vi "Write to Data Source.vi"(8 "error in (no error)":errorcluster, 11 "Projects in":refnum<class "Projects.lvclass">) -> (0 "error out":errorcluster, 3 "Projects out":refnum<class "Projects.lvclass">)   [LabVIEW 2020, in "Projects.lvclass"]
doc: "Write the data currently in the Project class data to the data source.\n\n03/2025 Erich Schlieper"
uses:
  Projects.lvclass
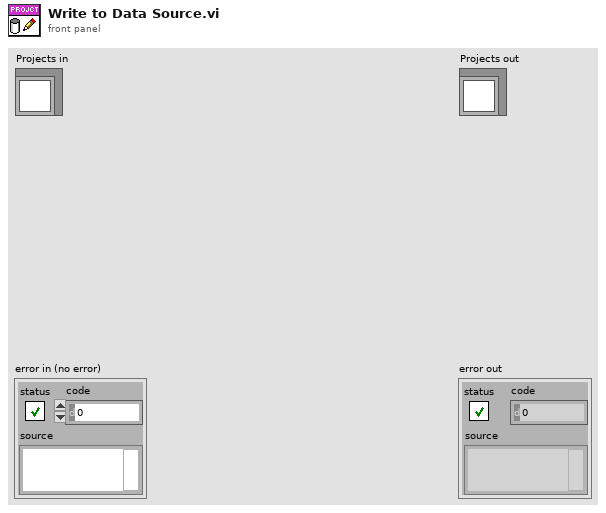
[diagram p1: front panel]
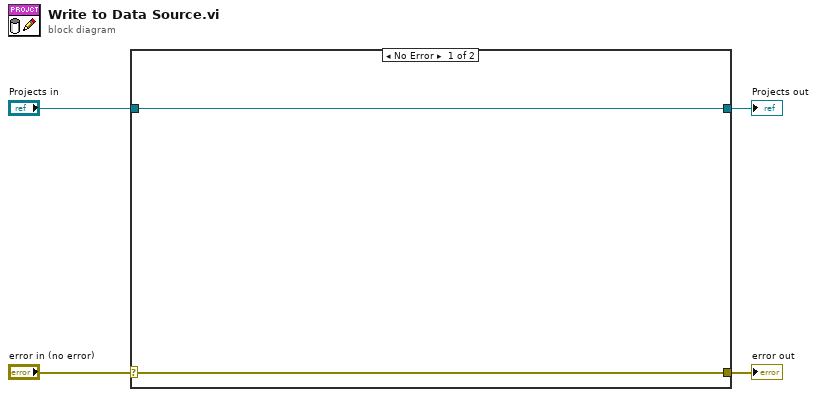
[diagram p0: block diagram]
diagram:
  n1 = case shown="No Error" "error in (no error)" {
    selector: "error in (no error)" -> [w5 w8]
    tunnel: [w5 w8] -> w3
    tunnel: [w6 w7] -> w1
    tunnel: "Projects in" -> [w6 w7]
    frame No Error {
    }
    frame Error {
    }
  }
  "error out" <- w3
  "Projects out" <- w1
